vi "MPDSnC Terminal Test.vi"() -> ()   [LabVIEW 2016]
uses:
  <vilib>/Instr/_visa.llb/VISA Configure Serial Port (Instr).vi
panel:
  out "Response":string
  in  "Quit":bool
  in  "Send Command":bool
  in  "Command":string
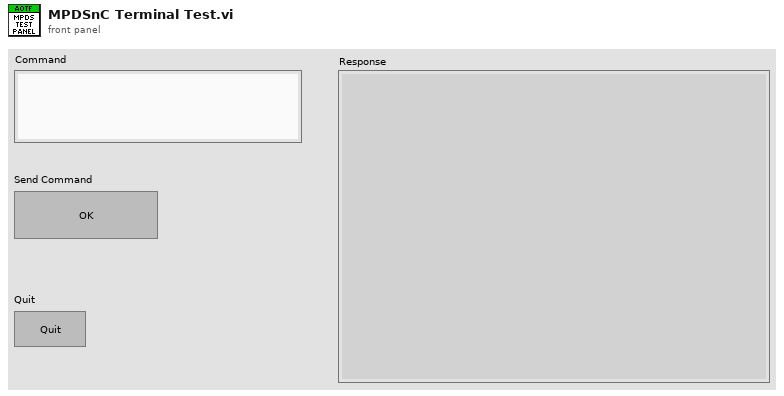
[diagram p1: front panel]
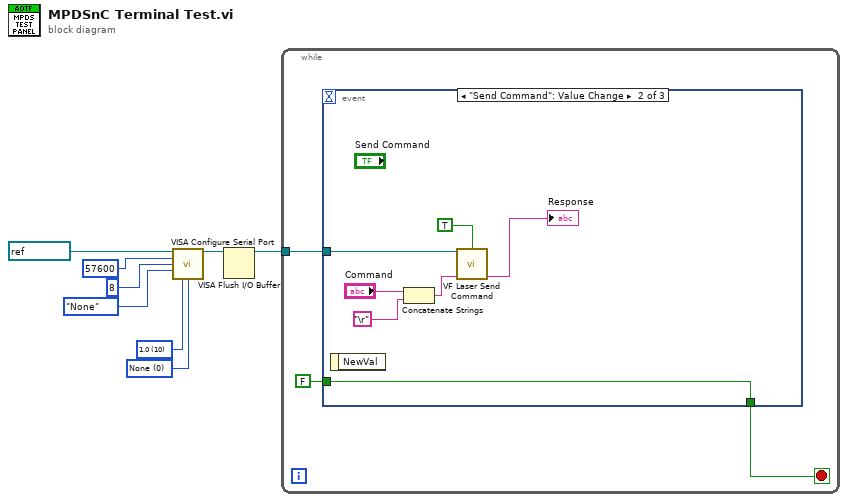
[diagram p0: block diagram]
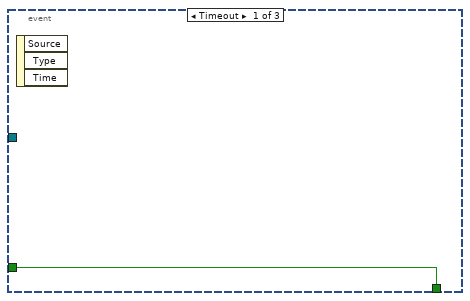
[diagram p2: hidden frame]
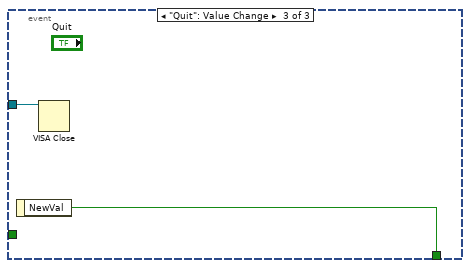
[diagram p3: hidden frame]
diagram:
  w8 = u16 0 items=["None", "XON/XOFF", "RTS/CTS", "XON/XOFF & RTS/CTS", "DTR/DSR", "XON/XOFF & DTR/DSR"] ("flow control (0:none)")
  w7 = u16 10 items=["1.0"=10, "1.5"=15, "2.0"=20] ("stop bits (10: 1 bit)")
  n1 = call-poly "VISA Configure Serial Port"("VISA resource name"=refnum<visa-resource-name> "COM6" ("reference"), "baud rate (9600)"=u32 57600, "data bits (8)"=u16 8, "parity (0:none)"=enum16{"None", "Odd", "Even", "Mark", "Space"}."None", "stop bits (10: 1 bit)"=w7, "flow control (0:none)"=w8) -> ("VISA resource name out"=w3:refnum<visa-resource-name>)  [unwired: 8 in, 1 out]
  n2 = VISA Flush I/O Buffer(VISA resource name=w3) -> (VISA resource name out=w2:refnum<visa-resource-name>)  [unwired: 2 in, 1 out]
  n3 = while {
    tunnel: w2 -> [w9]
    stop <- w11 stop-if-true
    n4 = event shown="[1] \"Send Command\": Value Change" {
      selector: _ -> [_ _ _]
      dyn-events: _ -> [_ _ _]
      timeout: _ -> [_ _ _]
      tunnel: [w12 w19 w21] -> w11
      tunnel: FALSE -> [w12 w19 _]
      tunnel: w9 -> [_ w18 w20]
      event Timeout {
        n5 = event-data() -> ()  [unwired: 1 in, 3 out]
      }
      event "Send Command": Value Change {
        n6 = event-data() -> ()  [unwired: 1 in, 1 out]
        n7 = Concatenate Strings("Command", "\r") -> (w14:string)
        n8 = call "VF Laser Send Command.vi"("VISA Ref"=w18, "Wait for Reply?"=TRUE, "Command"=w14) -> ("Response"=→"Response":string)  [unwired: 10 in, 2 out]
      }
      event "Quit": Value Change {
        n9 = event-data() -> ("NewVal"=w21:bool)  [unwired: 1 in]
        n10 = VISA Close(VISA resource name=w20) -> ()  [unwired: 1 in, 1 out]
      }
    }
  }
